vi "Set Cursor.vi"(8 "error in (no error)":errorcluster, 10 "position":cluster{"row":i8, "column":i8}, 11 "HD44780 in":refnum<class "HD44780.lvclass">) -> (0 "error out":errorcluster, 3 "HD44780 out":refnum<class "HD44780.lvclass">)   [LabVIEW 2017, in "HD44780.lvclass"]
uses:
  HD44780.lvclass
  HD44780.lvclass/HD44780.ctl
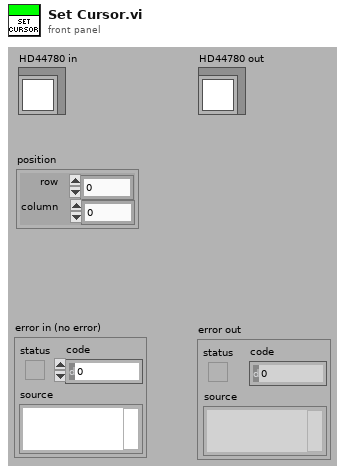
[diagram p1: front panel]
types:
  T1 = typedef "HD44780 Common.lvlib/cluster of class private data.ctl" = cluster{"FPGA VI Reference":refnum<k20>, "device index":i8, "screen size":T2, "font size":T3, "auto wrap":bool, "alignment":T4, "number of line":T5, "shift 0":i8, "entry mode 0":T6, "shift 1":i8, "entry mode 1":T6}
  T2 = typedef "HD44780 Common.lvlib/screen size.ctl" = enum8{"8x1", "8x2", "12x4", "16x1", "16x2", "16x4", "20x1", "20x2", "20x4", "24x1", "24x2", "40x2", "40x4"}
  T3 = typedef "HD44780 Common.lvlib/font size.ctl" = enum8{"5x8", "5x10"}
  T4 = typedef "HD44780 Common.lvlib/alignment.ctl" = enum16{"None", "Left", "Center", "Right"}
  T5 = typedef "HD44780 Common.lvlib/line number.ctl" = enum8{"1 line", "2 lines"}
  T6 = typedef "HD44780 Common.lvlib/entry mode.ctl" = enum8{"increment & no shift", "increment & shift", "decrement & no shift", "decrement & shift"}
  T7 = cluster{"FPGA VI Reference":refnum<k20>, "device index":i8, "screen size":enum8{"8x1", "8x2", "12x4", "16x1", "16x2", "16x4", "20x1", "20x2", "20x4", "24x1", "24x2", "40x2", "40x4"}, "font size":enum8{"5x8", "5x10"}, "auto wrap":bool, "alignment":enum16{"None", "Left", "Center", "Right"}, "number of line":enum8{"1 line", "2 lines"}, "shift 0":i8, "entry mode 0":enum8{"increment & no shift", "increment & shift", "decrement & no shift", "decrement & shift"}, "shift 1":i8, "entry mode 1":enum8{"increment & no shift", "increment & shift", "decrement & no shift", "decrement & shift"}}
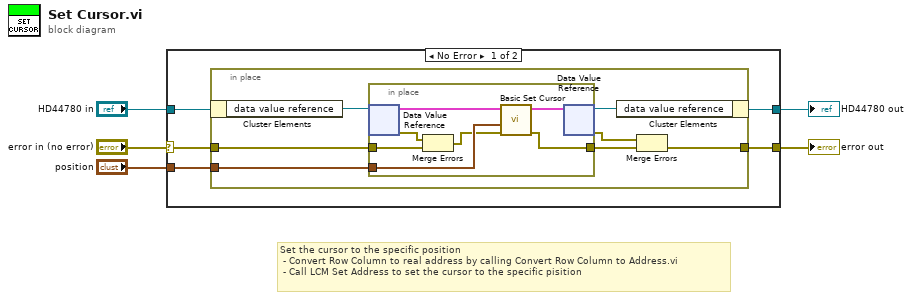
[diagram p0: block diagram]
diagram:
  # "Set the cursor to the specific position\n - Convert Row Column to real address by calling Convert Row Column to Address.vi \n - Call LCM Set Address to set the cursor to the specific pisition"
  n1 = case shown="No Error" "error in (no error)" {
    selector: "error in (no error)" -> [w8 w26]
    tunnel: [w9 w26] -> w4
    tunnel: "HD44780 in" -> [w7 w25]
    tunnel: "position" -> [w10 _]
    tunnel: [w6 w25] -> w1
    frame No Error {
      n2 = in-place {
        in-place-border: w10 -> [w17]
        in-place-border: [w14] -> w9
        in-place-border: w8 -> [w13]
        n3 = in-place-cluster #1(w7) -> ("data value reference"=w12:refnum<data-value>)
        n4 = in-place {
          in-place-border: w17 -> [w24]
          in-place-border: [w23] -> w15
          in-place-border: w13 -> [w20]
          n5 = in-place-dvr #2(w12) -> (w19:T1, w21:errorcluster)
          n6 = Merge Errors(w21, w20) -> (w18:errorcluster)
          n7 = call "Basic Set Cursor.vi"("error in (no error)"=w18, "position"=w24, "cluster of private data"=w19) -> ("error out"=w23:errorcluster, "cluster of private data out"=w22:T7)  [unwired: 6 in, 1 out]
          n8 = in-place-dvr #2(w22) -> (w11:refnum<data-value>, w16:errorcluster)
        }
        n9 = in-place-cluster #1("data value reference"=w11) -> (w6:refnum<class "HD44780.lvclass">)
        n10 = Merge Errors(w16, w15) -> (w14:errorcluster)
      }
    }
    frame Error {
    }
  }
  "error out" <- w4
  "HD44780 out" <- w1
